vi "TDMS_to_CSV_loop.vi"() -> ()   [LabVIEW 2012]
doc: "Reads a TDMS (Technical Data Management Streaming) file."
uses:
  <vilib>/Waveform/WDTOps.llb/WDT Get Waveform Time Array DBL.vi
panel:
  in  "error in":errorcluster
  in  "append to file? (new file:F)":bool
  in  "prompt":string
  out "Number of Channels":i32
  out "wf increment":dbl
  out "wf samples":i32
  out "Number of Samples":i32
  in  "#Samples to Process [Window]":i32=1000000
  out "Start Time Date":variant
  out "All Property values":variant[](array[variant])
  out "group/channel names":string[][](array[string])
  out "?":variant[](array[variant])
  out "?":string[](array[string])
  out "Waveform Graph":waveform(dbl)[](graph)
  # "Will average the values based on a window of a TDMS file. Will then print that to CSV. This is locked to 3 channels."
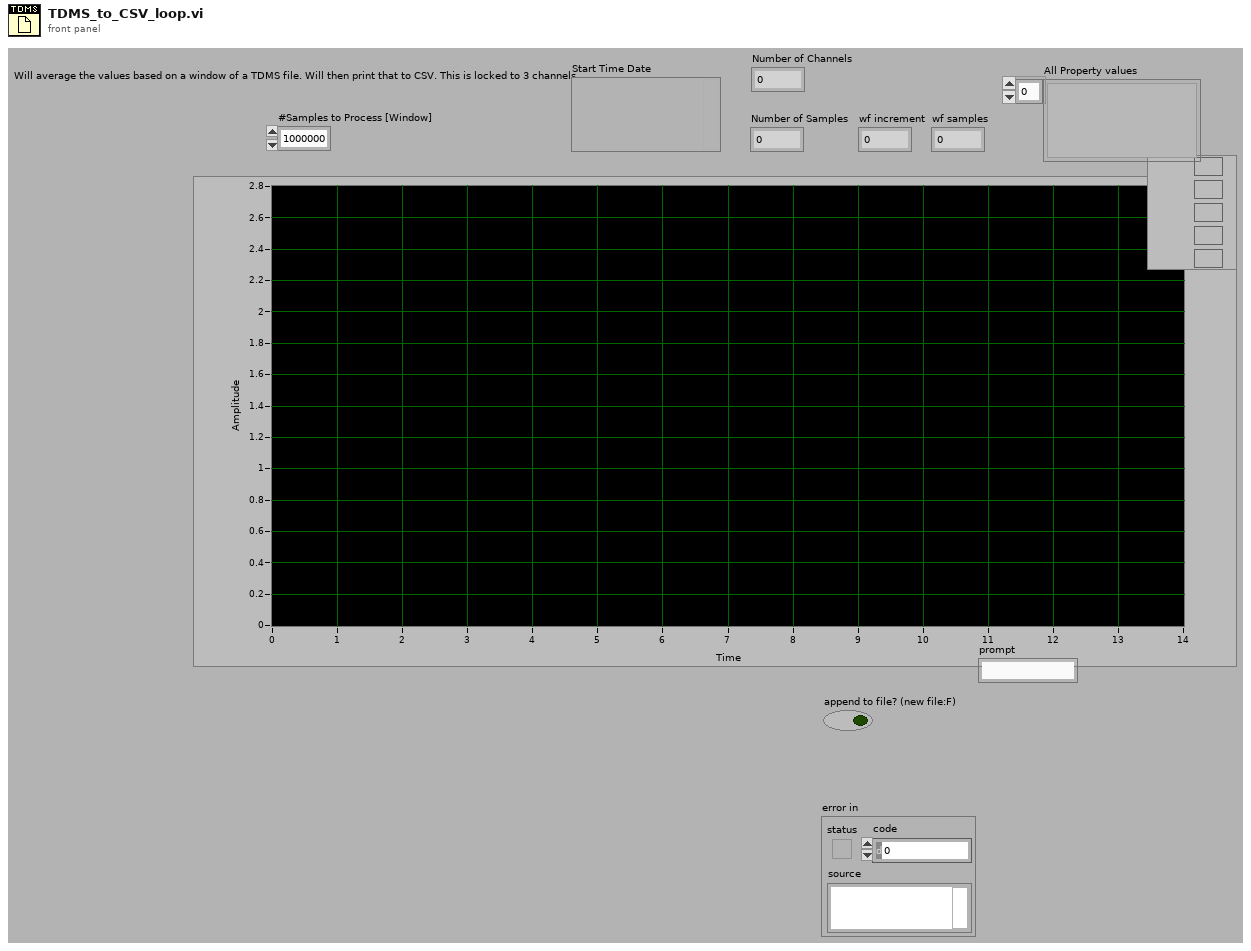
[diagram p1: front panel]
types:
  T1 = enum16{"open", "open or create", "create or replace", "create", "open (read-only)"}
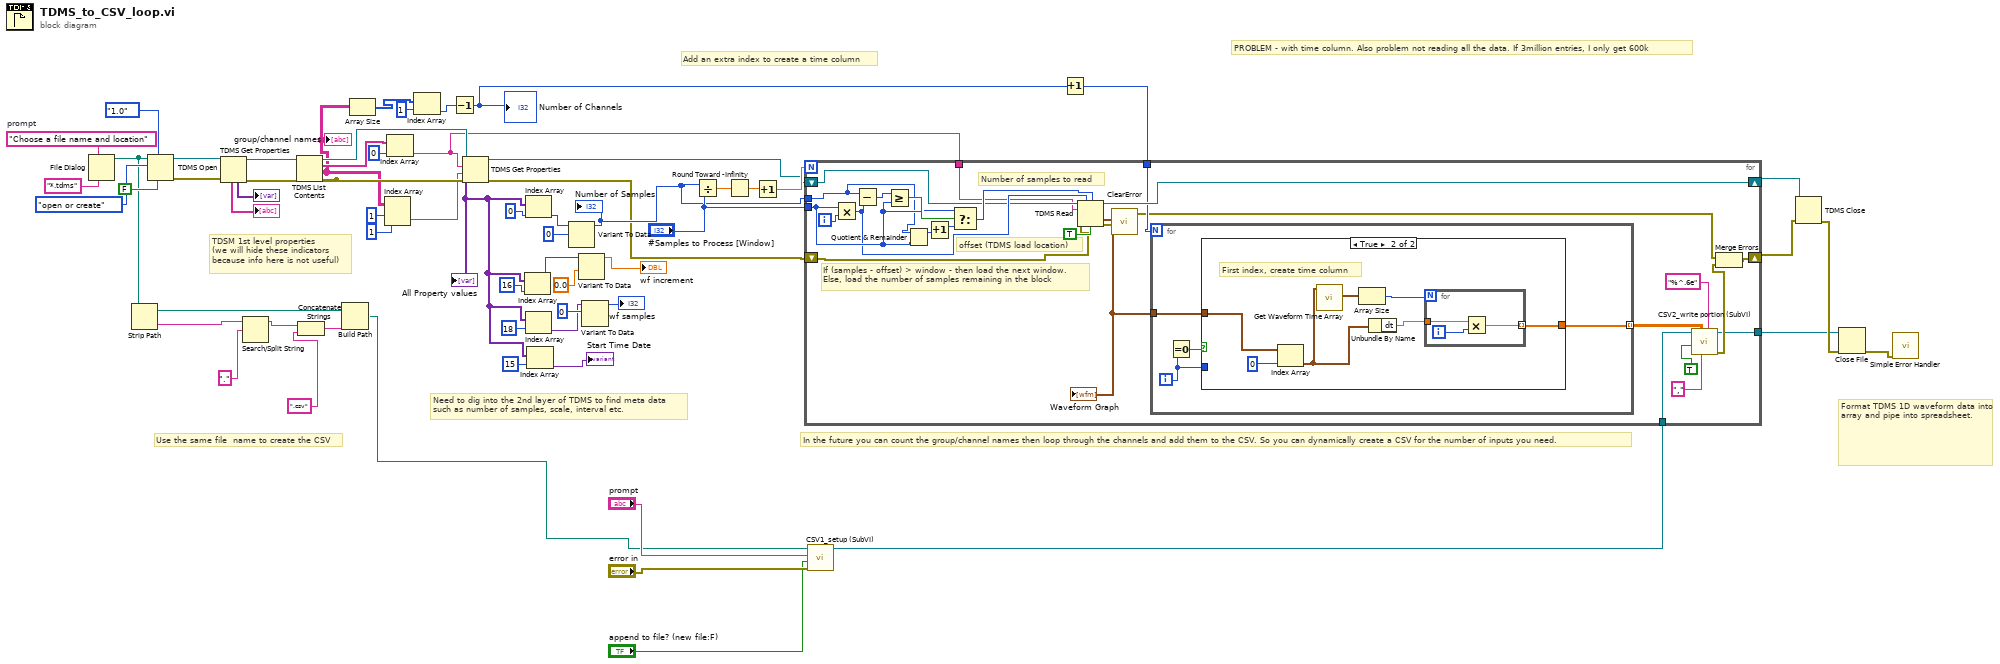
[diagram p0: block diagram]
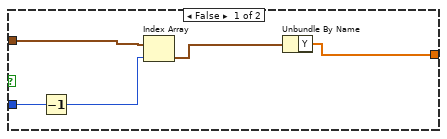
[diagram p2: hidden frame]
diagram:
  w62 = "Choose a file name and location"  # prompt
  # "PROBLEM - with time column. Also problem not reading all the data. If 3million entries, I only get 600k"
  # "Add an extra index to create a time column"
  # "Format TDMS 1D waveform data into array and pipe into spreadsheet."
  # "Use the same file  name to create the CSV"
  # "In the future you can count the group/channel names then loop through the channels and add them to the CSV. So you can dynamically create a CSV for the number of inputs you need."
  # "Need to dig into the 2nd layer of TDMS to find meta data\nsuch as number of samples, scale, interval etc."
  # "TDSM 1st level properties\n(we will hide these indicators\nbecause info here is not useful)"
  n1 = File Dialog(6:"*.tdms" ("pattern (all files)"), 7:w62) -> (3:w11:path)  [unwired: 1 in, 7 out]
  n2 = Strip Path(path=w11) -> (stripped path=w13:path, name=w17:string)
  n3 = TDMS Open(6:FALSE ("disable buffering (T)"), 7:enum16{"1.0", "2.0"}."1.0" ("file format version (2.0)"), 10:T1."open or create" ("operation"), 11:w11) -> (0:w55:errorcluster, 3:w54:refnum<k34>)  [unwired: 2 in]
  n4 = TDMS Get Properties(8:w55, 11:w54) -> (0:w52:errorcluster, 3:w53:refnum<k34>, 4:→"?":variant[], 6:→"?":string[])  [unwired: 6 out]
  n5 = Search/Split String(string=w17, search string/char (-)=".") -> (substring before match=w15:string)  [unwired: 1 in, 2 out]
  n6 = TDMS List Contents(4:w52, 7:w53) -> (1:w21:string[][], 2:w49:string[], 3:w46:refnum<k34>)  [unwired: 2 out]
  "group/channel names" <- w21
  n7 = Concatenate Strings(w15, ".csv" ("string")) -> (w12:string)
  n8 = Build Path(base path=w13, name or relative path=w12) -> (appended path=w3:path)
  n9 = Array Size(array=w21) -> (size(s)=w20:i32[])
  n10 = Index Array(array=w21, index (row)=1, index (col)=1 ("disabled index (col)")) -> (element=w47:string)
  n11 = Index Array(array=w49, index=0) -> (element=w29:string)
  n12 = Index Array(array=w20, index=1) -> (element=w18:i32)
  n13 = Decrement(x=w18) -> (x-1=w10:i32)
  "Number of Channels" <- w10
  n14 = TDMS Get Properties(8:w52, 9:w47, 10:w29, 11:w46) -> (0:w30:errorcluster, 3:w31:refnum<k34>, 4:w41:variant[])  [unwired: 5 out]
  "All Property values" <- w41
  n15 = Index Array(array=w41, index=16) -> (element=w27:variant)
  n16 = Index Array(array=w41, index=0) -> (element=w33:variant)
  n17 = Index Array(array=w41, index=18) -> (element=w26:variant)
  n18 = Index Array(array=w41, index=15) -> (element=→"Start Time Date":variant)
  n19 = Variant To Data(type=0, Variant=w33) -> (data=w32:i32)  [unwired: 1 in, 1 out]
  "Number of Samples" <- w32
  n20 = Variant To Data(type=0.0, Variant=w27) -> (data=→"wf increment":dbl)  [unwired: 1 in, 1 out]
  n21 = Variant To Data(type=0, Variant=w26) -> (data=→"wf samples":i32)  [unwired: 1 in, 1 out]
  n22 = Divide(x=w32, y="#Samples to Process [Window]") -> (x/y=w40:dbl)
  n23 = Round Toward -Infinity(1:w40) -> (0:w39:dbl)
  n24 = Increment(x=w39) -> (x+1=w38:dbl)
  n25 = call "CSV1_setup (SubVI).vi"("error in (no error)"="error in", "append to file? (new file:F)"="append to file? (new file:F)", "prompt"="prompt", "file path (dialog if empty)"=w3) -> ("file refnum out"=w2:refnum<file>)  [unwired: 6 in, 1 out]
  n26 = Increment(x=w10) -> (x+1=w9:i32)
  n27 = for {
    N: w38 -> [_]
    tunnel: "#Samples to Process [Window]" -> [w84]
    tunnel: w32 -> [w83]
    shift-right: [w77] -> w36
    shift-left: w31 -> [w76]
    shift-right: [w71] -> w35
    shift-left: w30 -> [w75]
    tunnel: w29 -> [w74]
    tunnel: w9 -> [w72]
    tunnel: w2 -> [w64]
    tunnel: [w63] -> w1
    i -> [w87]
    # "Number of samples to read"
    # "offset (TDMS load location)"
    # "If (samples - offset) > window - then load the next window.\nElse, load the number of samples remaining in the block"
    n28 = Multiply(x=w84, y=w87) -> (x*y=w78:i32)
    n29 = Subtract(x=w83, y=w78) -> (x-y=w86:i32)
    n30 = Greater Or Equal?(x=w86, y=w84) -> (x >= y?=w85:bool)
    n31 = Quotient & Remainder(x=w83, y=w84) -> (x-y*floor(x/y)=w81:i32)  [unwired: 1 out]
    n32 = Increment(x=w81) -> (x+1=w82:i32)
    n33 = Select(t=w84, s=w85, f=w82) -> (s? t:f=w79:i32)
    n34 = TDMS Read(0:w76, 1:w78, 2:w79, 5:w74, 11:w75, 13:TRUE ("return channels in file order? (F)")) -> (4:w77:refnum<k34>, 10:w73:waveform(dbl)[], 15:w70:errorcluster)  [unwired: 2 in, 3 out]
    "Waveform Graph" <- w73
    n35 = call <vilib>:"ClearError.vi"("error in (no error)"=w70) -> ()  [unwired: 1 out]
    n36 = for {
      N: w72 -> [_]
      tunnel: [w90] -> w65 mode=indexing
      tunnel: w73 -> [w89]
      i -> [w88]
      n37 = Equal To 0?(x=w88) -> (x = 0?=w91:bool)
      n38 = case shown="True" w91 {
        tunnel: [w95 w100] -> w90
        tunnel: w89 -> [w96 w97]
        tunnel: w88 -> [w92 _]
        frame False {
          n39 = Decrement(x=w92) -> (x-1=w93:i32)
          n40 = Index Array(array=w96, index=w93) -> (element=w94:waveform(dbl))
          n41 = Unbundle By Name(w94) -> ("Y"=w95:dbl[])
        }
        frame True {
          # "First index, create time column"
          n42 = Index Array(array=w97, index=0) -> (element=w99:waveform(dbl))
          n43 = call-poly <vilib>:"Get Waveform Time Array.vi"("waveform in"=w99) -> ("X array"=w103:timestamp[])  [unwired: 9 in, 1 out]
          n44 = Array Size(array=w103) -> (size(s)=w101:i32)
          n45 = Unbundle By Name(w99) -> ("dt"=w102:dbl)
          n46 = for {
            N: w101 -> [_]
            tunnel: w102 -> [w106]
            tunnel: [w104] -> w100 mode=indexing
            i -> [w105]
            n47 = Multiply(x=w106, y=w105) -> (x*y=w104:dbl)
          }
        }
      }
    }
    n48 = call "CSV2_write portion (SubVI).vi"("format (%.3f)"="%^.6e", "delimiter (\\t)"=",", "2D data"=w65, "transpose? (no:F)"=TRUE, "File Refnum in"=w64) -> ("error out"=w66:errorcluster, "File Refnum out"=w63:refnum<file>)  [unwired: 5 in]
    n49 = Merge Errors(w70, w66) -> (w71:errorcluster)
  }
  n50 = TDMS Close(8:w35, 11:w36) -> (0:w8:errorcluster)  [unwired: 1 out]
  n51 = Close File(refnum=w1, error in=w8) -> (error out=w7:errorcluster)  [unwired: 1 out]
  n52 = call <vilib>:"Simple Error Handler.vi"("error in (no error)"=w7) -> ()  [unwired: 1 in, 8 out]
